vi "Serial Write.vi"(8 "error in (no error)":errorcluster, 9 "Data":string, 10 "Node In":string, 11 "VISA resource name":refnum<visa-resource-name>) -> (0 "error out":errorcluster, 2 "Node Out":string, 3 "VISA resource name out":refnum<visa-resource-name>, 4 "Command String":string)   [LabVIEW 2012, in "Keithley 2600 Series.lvlib"]
doc: "This VI writes data to the instrument's RS-232 serial port.\n\nThis function will write the given string to the serial port where it can be read by equipment (e.g., component handler) connected to the other end of the serial port. No terminator characters are added to the data. The data will be written exactly as is.\n\n<b>Functions and Attributes Used</b>\nserial.write(data)\ndata - Specify the data string to write."
uses:
  Keithley 2600 Series.lvlib
  Private/GlobalVariables.vi
panel:
  # "(c) 2008 Keithley Instruments, Inc.  ALL RIGHTS RESERVED."
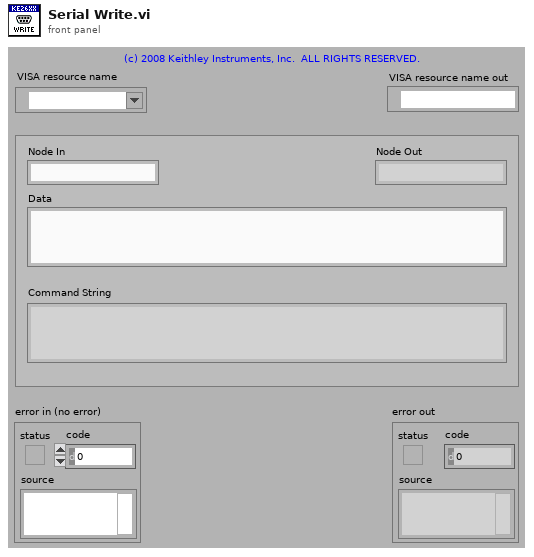
[diagram p1: front panel]
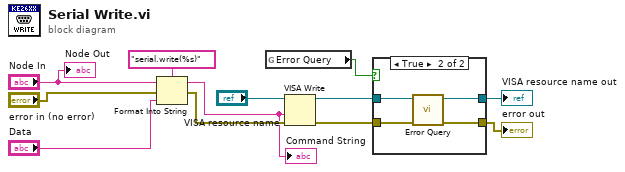
[diagram p0: block diagram]
diagram:
  n1 = Format Into String(format string="serial.write(%s)", initial string="Node In", error in="error in (no error)", "Data") -> (resulting string=w1:string, error out=w2:errorcluster)
  "Command String" <- w1
  n2 = global read "GlobalVariables.vi" "Error Query"() -> (w12:bool)
  n3 = VISA Write(VISA resource name="VISA resource name", write buffer=w1, error in (no error)=w2) -> (VISA resource name out=w11:refnum<visa-resource-name>, error out=w10:errorcluster)  [unwired: 1 out]
  n4 = case shown="True" w12 {
    tunnel: w11 -> [w14 w17]
    tunnel: w10 -> [w13 w18]
    tunnel: [w14 w16] -> w9
    tunnel: [w13 w15] -> w8
    frame False {
    }
    frame True {
      n5 = call "Error Query.vi"("error in (no error)"=w18, "VISA resource name"=w17) -> ("error out"=w15:errorcluster, "VISA resource name out"=w16:refnum<visa-resource-name>)  [unwired: 8 out]
    }
  }
  "VISA resource name out" <- w9
  "error out" <- w8
  "Node Out" <- "Node In"
